vi "Set Data Call Alg Get Data.vi"(4 "QWTB Folder Path":path=path "", 5 "Calculation Settings":T2={"Strict"=FALSE, "Verbose"=TRUE, "Uncertainty Calculation Method"=enum."none", "Correlations"={"Required"=FALSE, "Generate"=FALSE}, "Degrees of Freedom"={"Required"=FALSE, "Generate"=FALSE}, "MCM Calculation Settings"={"Repeats"=100, "Verbose"=TRUE, "Parallelization method"=enum."Single Core", "Processors"=0, "Temporary directory"=".", "Randomize"=TRUE}} {"MCM Calculation Settings"."Processors" min=0 step=1; "MCM Calculation Settings"."Repeats" min=1 step=1}, 6 "Backend engine":T8, 7 "Algorithm ID":string, 8 "error in":errorcluster, 11 "Data In":T1[](array[typedef])=[{"Name"="", "Value"=[], "Uncertainty"=[], "Degrees of Freedom"=[], "Correlation"=[], "Randomized uncertainty"=[]}]) -> (0 "error out":errorcluster, 1 "qwtb.m found in path":bool, 3 "Data Out":T1[](array[typedef]))   [LabVIEW 2013, in "QWTBLVLib.lvlib"]
doc: "Clears Matlab variables, set working path, writes input data, writes calculation settings, calls algorithm, reads output data."
uses:
  QWTBLVLib.lvlib
  TD Quantity.ctl
  TD Backend Engine.ctl
  TD Calculation Settings.ctl
  TD Uncertainty Calculation Method.ctl
  TD Correlation Calculation Settings.ctl
  TD DOF Calculation Settings.ctl
  TD MCM Calculation Settings.ctl
  TD MCM Calculation Method.ctl
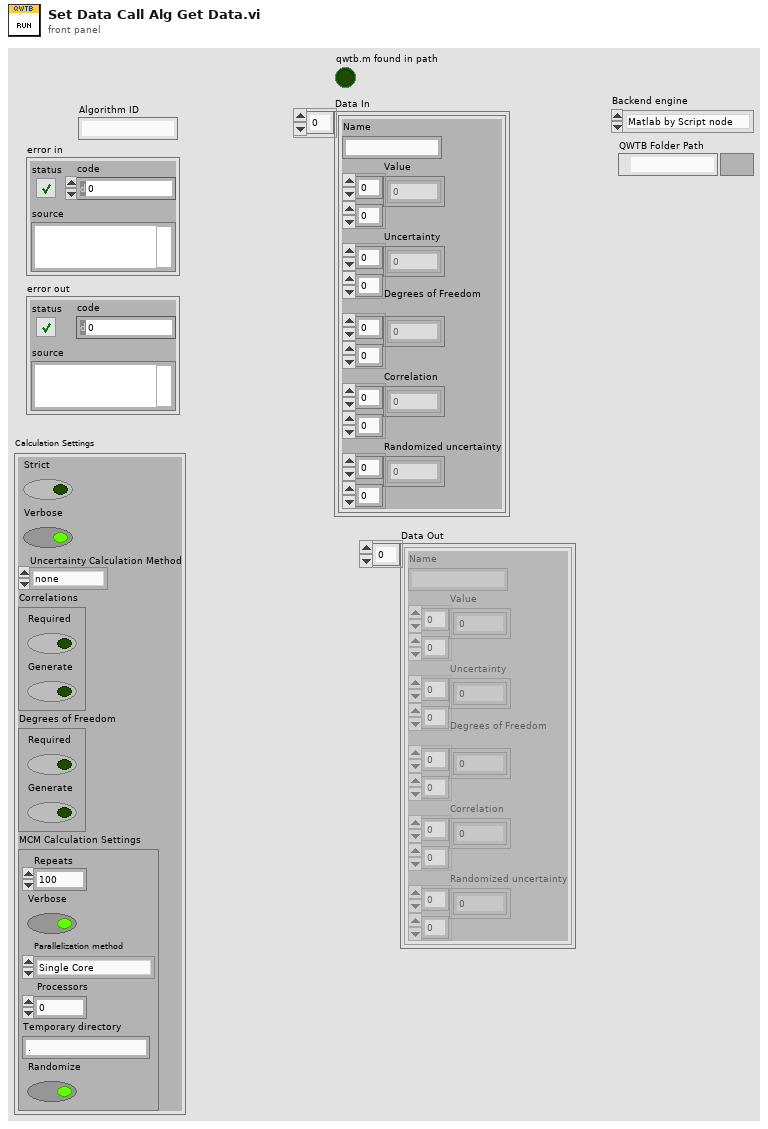
[diagram p1: front panel]
types:
  T1 = typedef "QWTBLVLib.lvlib/TD Quantity.ctl" = cluster{"Name":string, "Value":dbl[][], "Uncertainty":dbl[][], "Degrees of Freedom":dbl[][], "Correlation":dbl[][], "Randomized uncertainty":dbl[][]}
  T2 = typedef "QWTBLVLib.lvlib/TD Calculation Settings.ctl" = cluster{"Strict":bool, "Verbose":bool, "Uncertainty Calculation Method":T3, "Correlations":T4, "Degrees of Freedom":T5, "MCM Calculation Settings":T6}
  T3 = typedef "QWTBLVLib.lvlib/TD Uncertainty Calculation Method.ctl" = enum16{"none", "GUF", "MCM"}
  T4 = typedef "QWTBLVLib.lvlib/TD Correlation Calculation Settings.ctl" = cluster{"Required":bool, "Generate":bool}
  T5 = typedef "QWTBLVLib.lvlib/TD DOF Calculation Settings.ctl" = cluster{"Required":bool, "Generate":bool}
  T6 = typedef "QWTBLVLib.lvlib/TD MCM Calculation Settings.ctl" = cluster{"Repeats":i32, "Verbose":bool, "Parallelization method":T7, "Processors":i32, "Temporary directory":string, "Randomize":bool}
  T7 = typedef "QWTBLVLib.lvlib/TD MCM Calculation Method.ctl" = enum16{"Single Core", "Multi Core", "Multi Station"}
  T8 = typedef "QWTBLVLib.lvlib/TD Backend Engine.ctl" = enum16{"Matlab by Script node", "GNU Octave by GOLPI"}
  T9 = typedef "QWTBLVLib.lvlib/TD Algorithm Information.ctl" = cluster{"ID":string, "Name":string, "Description":string, "Citation":string, "Remarks":string, "License":string, "Inputs":T10[], "Outputs":T11[], "Provides GUF":bool, "Provides MCM":bool, "Full path":string}
  T10 = typedef "QWTBLVLib.lvlib/TD Algorithm Information Input.ctl" = cluster{"Name":string, "Description":string, "Alternative":i32, "Optional":i32, "Parameter":i32}
  T11 = typedef "QWTBLVLib.lvlib/TD Algorithm Information Output.ctl" = cluster{"Name":string, "Description":string}
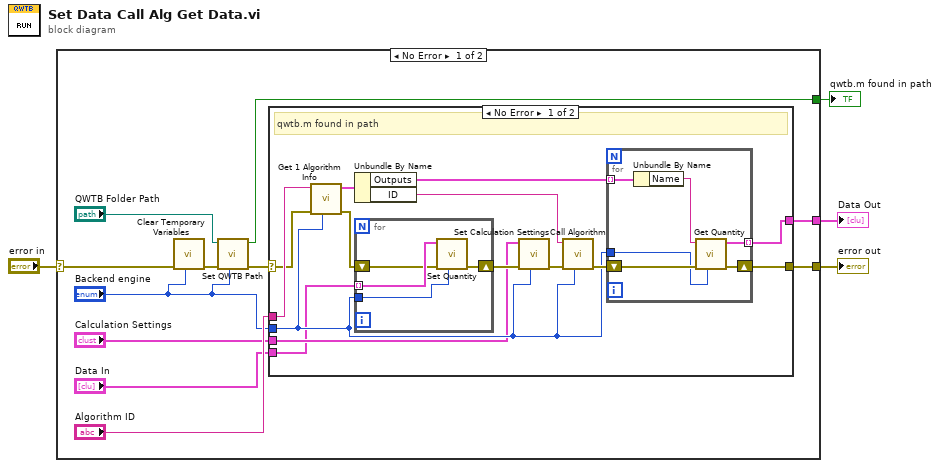
[diagram p0: block diagram]
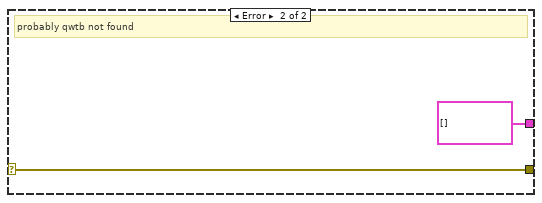
[diagram p2: hidden frame]
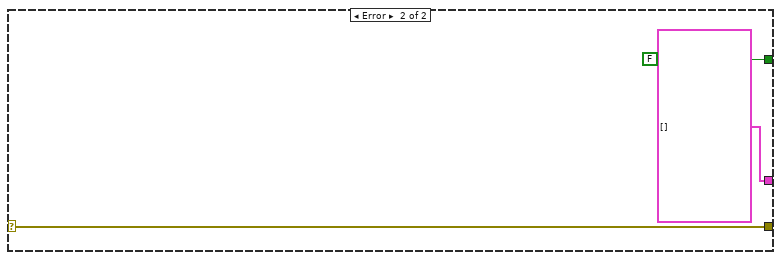
[diagram p3: hidden frame]
diagram:
  n1 = case shown="No Error" "error in" {
    selector: "error in" -> [w11 w44]
    tunnel: [w15 w44] -> w4
    tunnel: [w14 T1[] []] -> w2
    tunnel: [w5 FALSE ("qwtb.m found in path")] -> w1
    frame No Error {
      n2 = call "Clear Temporary Variables.vi"("Backend engine"="Backend engine", "error in"=w11) -> ("error out"=w12:errorcluster)  [unwired: 9 in]
      n3 = call "Set QWTB Path.vi"("Backend engine"="Backend engine", "error in"=w12, "QWTB Folder Path"="QWTB Folder Path") -> ("error out"=w6:errorcluster, "qwtb.m found in path"=w5:bool)  [unwired: 7 in]
      n4 = case shown="No Error" w6 {
        selector: w6 -> [w16 w40]
        tunnel: [w28 w40] -> w15
        tunnel: [w23 T1[] []] -> w14
        tunnel: "Algorithm ID" -> [w22 _]
        tunnel: "Backend engine" -> [w19 _]
        tunnel: "Calculation Settings" -> [w18 _]
        tunnel: "Data In" -> [w17 _]
        frame No Error {
          # "qwtb.m found in path"
          n5 = call "Get 1 Algorithm Info.vi"("Backend engine"=w19, "error in (no error)"=w16, "Algorithm ID"=w22) -> ("error out"=w20:errorcluster, "Algorithm Information"=w21:T9)  [unwired: 7 in]
          n6 = Unbundle By Name(w21) -> ("Outputs"=w25:T11[], "ID"=w24:string)
          n7 = for {
            tunnel: w17 -> [w39] mode=indexing
            shift-right: [w37] -> w27
            shift-left: w20 -> [w38]
            tunnel: w19 -> [w36]
            n8 = call "Set Quantity.vi"("Backend engine"=w36, "error in"=w38, "Quantity"=w39) -> ("error out"=w37:errorcluster)  [unwired: 8 in]
          }
          n9 = call "Set Calculation Settings.vi"("Backend engine"=w19, "error in"=w27, "Calculation Settings"=w18) -> ("error out"=w26:errorcluster)  [unwired: 8 in]
          n10 = call "Call Algorithm.vi"("Backend engine"=w19, "error in"=w26, "Algorithm ID"=w24) -> ("error out"=w29:errorcluster)  [unwired: 8 in]
          n11 = for {
            shift-right: [w34] -> w28
            shift-left: w29 -> [w35]
            tunnel: [w33] -> w23 mode=indexing
            tunnel: w25 -> [w31] mode=indexing
            tunnel: w19 -> [w32]
            n12 = Unbundle By Name(w31) -> ("Name"=w30:string)
            n13 = call "Get Quantity.vi"("Backend engine"=w32, "error in"=w35, "Quantity Name"=w30) -> ("error out"=w34:errorcluster, "Quantity"=w33:T1)  [unwired: 7 in]
          }
        }
        frame Error {
          # "probably qwtb not found"
        }
      }
    }
    frame Error {
    }
  }
  "error out" <- w4
  "Data Out" <- w2
  "qwtb.m found in path" <- w1
